vi "Open Device.vi"   [LabVIEW 2019, in "D2XX-lv.lvlib"]
doc: "Open the specified device and return a handle that will be used for subsequent accesses. The device can be specified by its serial number or index."
uses:
  D2XX-lv.lvlib
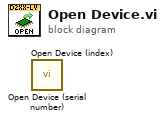
[diagram p0: block diagram]
diagram:
  n1 = call "Open Device (serial number).vi"() -> ()  [unwired: 10 in, 2 out]
  n2 = call "Open Device (index).vi"() -> ()  [unwired: 10 in, 2 out]
